vi "readFromXML.vi"(8 "error in (no error)":errorcluster, 10 "XML in":string, 11 "ADCPointingCorrectionOffsets in":refnum<class "ADCPointingCorrectionOffsets.lvclass">) -> (0 "error out":errorcluster, 3 "ADCPointingCorrectionOffsets out":refnum<class "ADCPointingCorrectionOffsets.lvclass">)   [LabVIEW 2014, in "TCSDataDefinitions.lvlib" / "TCSAtmosphericDispersionCommand.lvlib" / "ADCPointingCorrectionOffsets.lvclass"]
uses:
  ADCPointingCorrectionOffsets.lvclass
  <userlib>/Common/UnitsAndXML/FlattenItemWithUnitToXML/FlattenPlaneAngleToXML/PlaneAngleUnit.ctl
  ADCPointingCorrectionOffsets.lvclass/ADCPointingCorrectionOffsets.ctl
  TCSAtmosphericDispersionCommand/TCSAtmosphericDispersionCommand.lvclass
  <userlib>/Common/UnitsAndXML/UnitsAndXML.lvlib
  <userlib>/Common/XML/XMLParser/XMLParser.lvclass
panel:
  out "yPointingCorrection_arcsec":dbl[unit]
  out "xPointingCorrection_arcsec":dbl[unit]
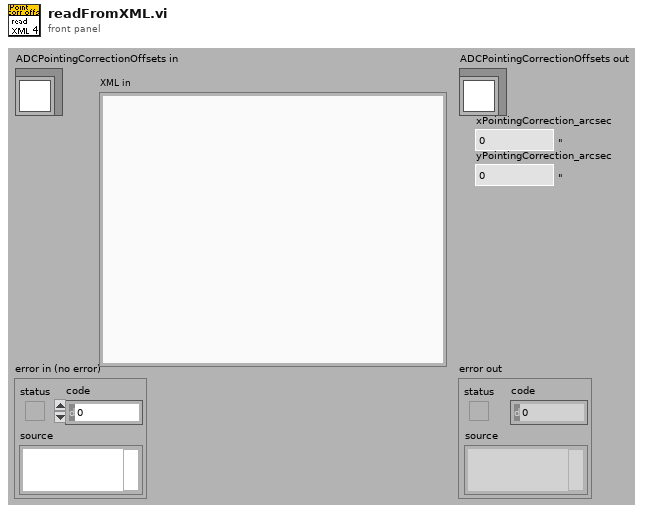
[diagram p1: front panel]
types:
  T1 = typedef "UnitsAndXML.lvlib/PlaneAngleUnit.ctl" = enum16{"rad", "deg", "'", "\""}
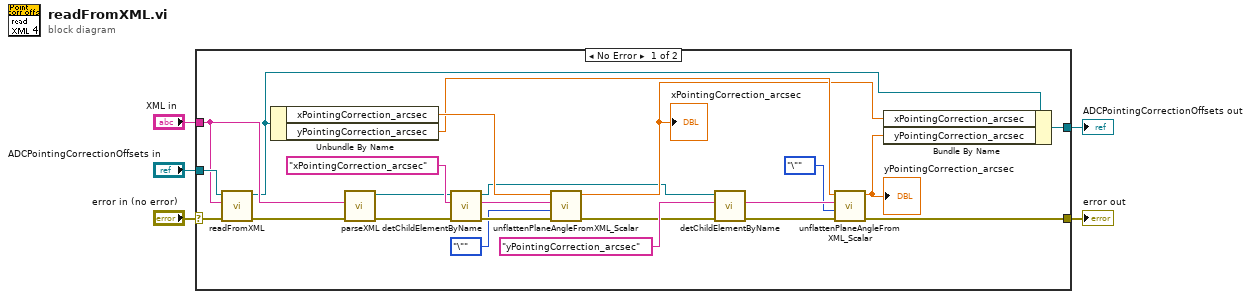
[diagram p0: block diagram]
diagram:
  n1 = case shown="No Error" "error in (no error)" {
    selector: "error in (no error)" -> [w23 w30]
    tunnel: [w9 w30] -> w4
    tunnel: [w20 w29] -> w2
    tunnel: "ADCPointingCorrectionOffsets in" -> [w25 w29]
    tunnel: "XML in" -> [w24 _]
    frame No Error {
      n2 = call-parent "readFromXML.vi"("error in (no error)"=w23, "XML in"=w24, "TCSAtmosphericDispersionCommand in"=w25) -> ("error out"=w22:errorcluster, "TCSAtmosphericDispersionCommand out"=w21:refnum<class "ADCPointingCorrectionOffsets.lvclass">)  [unwired: 7 out]
      n3 = Unbundle By Name(w21) -> ("xPointingCorrection_arcsec"=w17:dbl[unit], "yPointingCorrection_arcsec"=w12:dbl[unit])
      n4 = call <userlib>:"parseXML.vi"("error in (no error)"=w22, "XMLString in"=w24) -> ("error out"=w28:errorcluster, "Element out"=w7:refnum<class "XMLParser.lvclass">)  [unwired: 8 in]
      n5 = call <userlib>:"detChildElementByName.vi"("error in (no error)"=w28, "childName"="xPointingCorrection_arcsec" ("ChildName"), "Element in"=w7) -> ("error out"=w19:errorcluster, "childXML"=w18:string, "Element out"=w6:refnum<class "XMLParser.lvclass">)  [unwired: 5 in, 1 out]
      n6 = call <userlib>:"unflattenPlaneAngleFromXML_Scalar.vi"("error in (no error)"=w19, "planeAngleUnitInXML"=PlaneAngleUnit."\"", "xmlString"=w18, "planeAngleForType"=w17) -> ("error out"=w15:errorcluster, "planeAngle"=w11:dbl[unit])  [unwired: 6 in]
      "xPointingCorrection_arcsec" <- w11
      n7 = call <userlib>:"detChildElementByName.vi"("error in (no error)"=w15, "childName"="yPointingCorrection_arcsec" ("ChildName"), "Element in"=w6) -> ("error out"=w14:errorcluster, "childXML"=w13:string)  [unwired: 5 in, 2 out]
      n8 = call <userlib>:"unflattenPlaneAngleFromXML_Scalar.vi"("error in (no error)"=w14, "planeAngleUnitInXML"=PlaneAngleUnit."\"", "xmlString"=w13, "planeAngleForType"=w12) -> ("error out"=w9:errorcluster, "planeAngle"=w10:dbl[unit])  [unwired: 6 in]
      "yPointingCorrection_arcsec" <- w10
      n9 = Bundle By Name(cluster=w21, "xPointingCorrection_arcsec"=w11, "yPointingCorrection_arcsec"=w10) -> (w20:refnum<class "ADCPointingCorrectionOffsets.lvclass">)
    }
    frame Error {
    }
  }
  "error out" <- w4
  "ADCPointingCorrectionOffsets out" <- w2
